vi "Perform Data Limit File Operations.vi"(0 "VISA resource name":refnum<visa-resource-name>, 1 "Data File Operation (3: Save Limit Data File)":u16(ring)=3 items=["Delete Data File", "Delete All Data Files", "Recall Limit Data File", "Save Limit Data File"], 5 "Limit Line (1)":i32=1 min=1 max=6, 7 "Data Filename (TEST.xml)":string="TEST.xml", 9 "Driver Letter (D)":string="D", 11 "error in (no error)":errorcluster) -> (4 "VISA resource name out":refnum<visa-resource-name>, 15 "error out":errorcluster)   [LabVIEW 2020, in "Anritsu Signal Analyzer Series.lvlib"]
doc: "Deletes (Data file or all files), Recalls, or Saves the contents of the Limit data file."
uses:
  Anritsu Signal Analyzer Series.lvlib
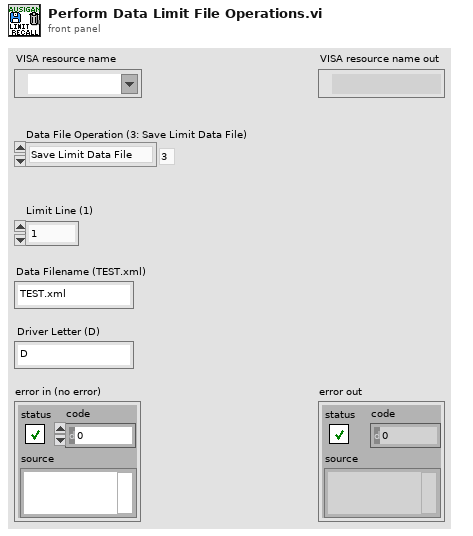
[diagram p1: front panel]
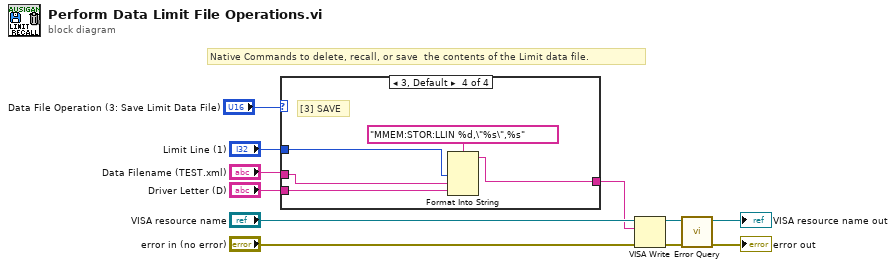
[diagram p0: block diagram]
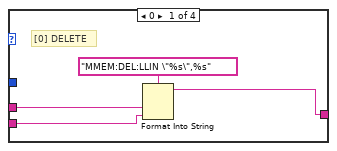
[diagram p2: hidden frame]
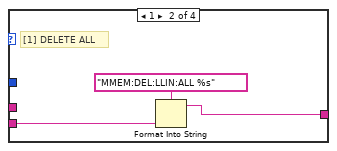
[diagram p3: hidden frame]
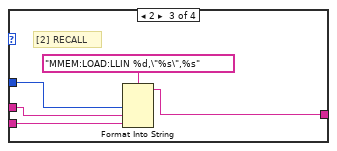
[diagram p4: hidden frame]
diagram:
  # "Native Commands to delete, recall, or save  the contents of the Limit data file."
  n1 = case shown="3, Default" "Data File Operation (3: Save Limit Data File)" {
    tunnel: "Data Filename (TEST.xml)" -> [w14 _ w23 w26]
    tunnel: "Driver Letter (D)" -> [w13 w17 w22 w25]
    tunnel: [w12 w16 w20 w24] -> w5
    tunnel: "Limit Line (1)" -> [_ _ w19 w27]
    frame 0 {
      # "[0] DELETE"
      n2 = Format Into String(format string="MMEM:DEL:LLIN \"%s\",%s" ("_Command"), w14, w13) -> (resulting string=w12:string)  [unwired: 2 in, 1 out]
    }
    frame 1 {
      # "[1] DELETE ALL"
      n3 = Format Into String(format string="MMEM:DEL:LLIN:ALL %s" ("_Command"), w17) -> (resulting string=w16:string)  [unwired: 2 in, 1 out]
    }
    frame 2 {
      # "[2] RECALL"
      n4 = Format Into String(format string="MMEM:LOAD:LLIN %d,\"%s\",%s" ("_Command"), w19, w23, w22) -> (resulting string=w20:string)  [unwired: 2 in, 1 out]
    }
    frame 3, Default {
      # "[3] SAVE"
      n5 = Format Into String(format string="MMEM:STOR:LLIN %d,\"%s\",%s" ("_Command"), w27, w26, w25) -> (resulting string=w24:string)  [unwired: 2 in, 1 out]
    }
  }
  n6 = VISA Write(VISA resource name="VISA resource name", write buffer=w5, error in (no error)="error in (no error)") -> (VISA resource name out=w3:refnum<visa-resource-name>, error out=w4:errorcluster)  [unwired: 1 out]
  n7 = call "Error Query.vi"("error in (no error)"=w4, "VISA resource name"=w3) -> ("error out"=→"error out":errorcluster, "VISA resource name out"=→"VISA resource name out":refnum<visa-resource-name>)  [unwired: 6 in, 2 out]
